vi "Receive Signal.vi"(8 "error in":errorcluster, 10 "Frame.Signal":string, 11 "PCAN in":refnum<class "PCAN.lvclass">) -> (0 "error out":errorcluster, 1 "Timestamp":timestamp format="%<%x %.3X>T", 2 "Value":dbl, 3 "PCAN out":refnum<class "PCAN.lvclass">)   [LabVIEW 2024, in "PCAN.lvlib" / "PCAN.lvclass"]
uses:
  PCAN.lvclass
  PCAN.lvclass/PCAN.ctl
  c6e083b5-7be6-46b7-8469-d6fd9ebf7a3d.vi
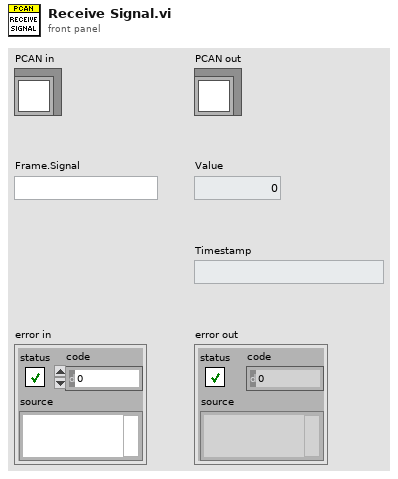
[diagram p1: front panel]
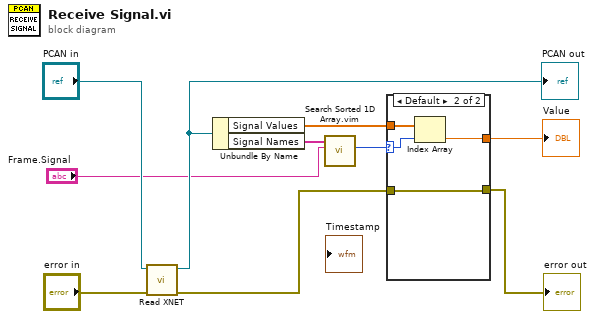
[diagram p0: block diagram]
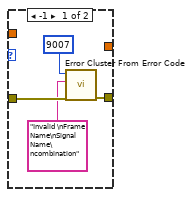
[diagram p2: hidden frame]
diagram:
  n1 = call "Read XNET.vi"("error in"="error in", "PCAN in"="PCAN in") -> ("error out"=w3:errorcluster, "PCAN out"=w8:refnum<class "PCAN.lvclass">)  [unwired: 8 in]
  "PCAN out" <- w8
  n2 = Unbundle By Name(w8) -> ("Signal Values"=w7:dbl[], "Signal Names"=w2:string[])
  n3 = call "Search Sorted 1D Array.vim"("element"="Frame.Signal", "sorted 1D array"=w2) -> ("nearest index"=w1:i32)  [unwired: 8 in, 1 out]
  n4 = case shown="Default" w1 {
    selector: w1 -> [_ w15]
    tunnel: w7 -> [_ w18]
    tunnel: [_ w17] -> w6
    tunnel: w3 -> [w14 w16]
    tunnel: [w13 w16] -> w5
    frame -1 {
      n5 = call <vilib>:"Error Cluster From Error Code.vi"("error in (no error)"=w14, "error message (\"\")"="Invalid \nFrame Name\nSignal Name\ncombination" ("error message (\"\")"), "error code (0)"=9007) -> ("error out"=w13:errorcluster)  [unwired: 6 in]
    }
    frame Default {
      n6 = Index Array(array=w18, index=w15) -> (element=w17:dbl)
    }
  }
  "error out" <- w5
  "Value" <- w6
